vi "Write To Spreadsheet File (DBL)2.vi"(0 "delimiter (\\t)":string="\t", 1 "transpose? (no:F)":bool, 4 "format (%.3f)":string="%.3f", 5 "append to file? (new file:F)":bool, 6 "1D data":dbl[](array[numeric]) format="%0.2f", 7 "2D data":dbl[][](array[numeric]) format="%0.2f", 8 "file path (dialog if empty)":path) -> (2 "error out":errorcluster, 3 "new file path (Not A Path if cancelled)":path)   [LabVIEW 2020]
doc: "LabVIEW no longer supports this VI. Use the Write Delimited Spreadsheet VI instead.\n\nConverts a 2D or 1D array of strings, signed integers, or double-precision numbers to a text string and writes the string to a new byte stream file or appends the string to an existing file. Wire data to the <B>2D data</B> input or <B>1D data</B> input to determine the polymorphic instance to use or manually select the instance.\n\nUse this VI to transpose or separate data.\n\n<B>Note</B> To format with Microsoft Excel, use ActiveX with LabVIEW or the Report Generation Toolkit for Microsoft Office.\n\nWhen you use this VI to transpose the data, the VI opens or creates the file before writing to it and closes it afterwards. You can use this VI to create a text file readable by most spreadsheet applications. This VI calls the Array To Spreadsheet String function to convert the data."
panel:
  in  "prompt":string="Choose file to write."
  # "This VI is deprecated. Use the following VI instead:\n\nvi.lib\\Utility\\file.llb\\Write Delimited Spreadsheet.vi"
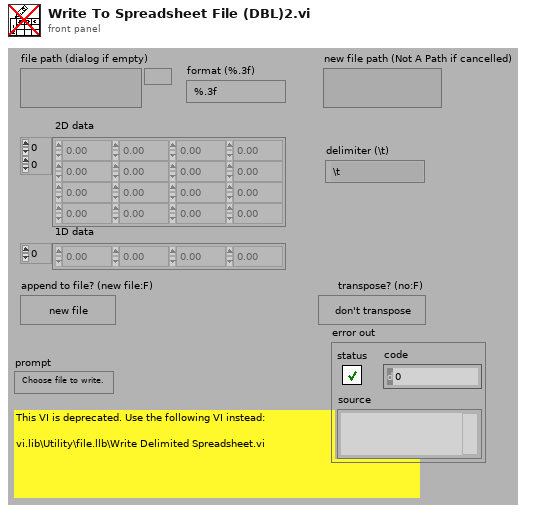
[diagram p1: front panel]
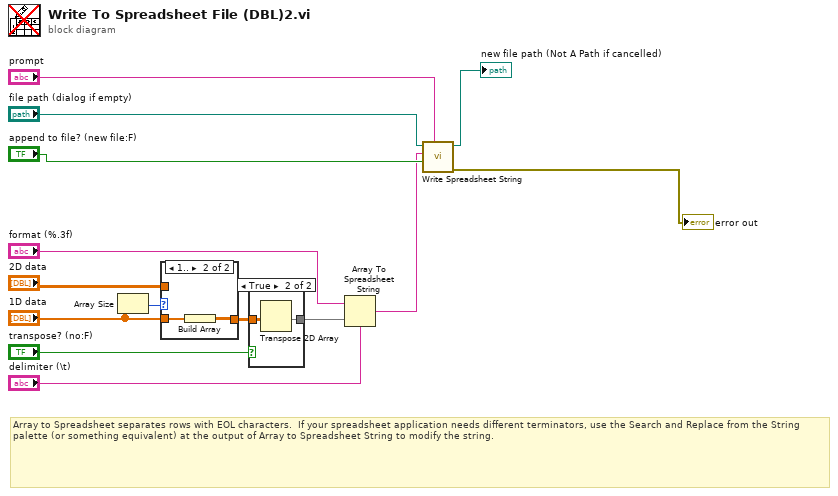
[diagram p0: block diagram]
diagram:
  # "Array to Spreadsheet separates rows with EOL characters.  If your spreadsheet application needs different terminators, use the Search and Replace from the String palette (or something equivalent) at the output of Array to Spreadsheet String to modify the string."
  n1 = Array Size(array="1D data") -> (size(s)=w13:i32)
  n2 = case shown="1.." w13 {
    tunnel: "1D data" -> [_ w17]
    tunnel: [w15 w16] -> w9
    tunnel: "2D data" -> [w15 _]
    frame ..0 {
      # "1D array is empty"
    }
    frame 1.. {
      n3 = Build Array(w17) -> (w16:dbl[][])
    }
  }
  n4 = case shown="True" "transpose? (no:F)" {
    tunnel: [w18 w20] -> w7
    tunnel: w9 -> [w18 w19]
    frame False {
    }
    frame True {
      n5 = Transpose 2D Array(2D array=w19) -> (transposed array=w20:dbl[][])
    }
  }
  n6 = Array To Spreadsheet String(delimiter (Tab)="delimiter (\\t)", array=w7, 3:"format (%.3f)") -> (spreadsheet string=w2:string)
  n7 = call <vilib>:"Write Spreadsheet String.vi"("prompt"="prompt", "append to file? (new file:F)"="append to file? (new file:F)", "spreadsheet string"=w2, "file path (dialog if empty)"="file path (dialog if empty)") -> ("error out"=→"error out":errorcluster, "path"=→"new file path (Not A Path if cancelled)":path)  [unwired: 6 in]
